vi "data.vi"() -> ()   [LabVIEW 2017]
panel:
  in  "data":dbl
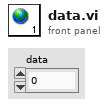
[diagram p1: front panel]
diagram:
